vi "DG Do Single Measurement.vi"(6 "Iteration index":i32, 7 "TWM handle in":i32, 8 "error in (no error)":errorcluster, 9 "DG measurement":T1={"Signal frequencies (Hz)"=[1000.0], "Signal amplitudes (V)"=[0.707], "Sampling frequencies (Hz)"=[10000000.0], "Record lengths (multiples of periods)"=[10000.0], "Calculate results"=FALSE, "Algorithm"="TWM-PJVSSubS", "TWM data directories"=[], "TWM data directories relative"=[], "PJVS frequencies (Hz)"=[1000.0], "PJVS reference voltages array of vector cluster"=[], "Requested PJVS steps"=[20], "Data folder"=path "", "Rs"=0, "Re"=0, "Settle down after PJVS change (s)"=1.0, "Switch position"=0.0, "PJVS amplitudes (Hz)"=[1000.0], "DG measurement info files"=[]} {"PJVS amplitudes (Hz)" format="%#_3p"; "PJVS reference voltages array of vector cluster"."PJVS reference voltages vector" format="%#_3p"; "PJVS frequencies (Hz)" format="%#_3p"; "Record lengths (multiples of periods)" format="%#_3p"; "Sampling frequencies (Hz)" format="%#_3p"; "Signal amplitudes (V)" format="%#_3p"; "Signal frequencies (Hz)" format="%#_3p"}, 10 "Common properties":T2={"Measurement status ref"=refnum, "TWM Status ref"=refnum, "Abort ref"=refnum, "Skip waiting ref"=refnum, "GNU Octave path"=path "C:/Program Files/GNU Octave/Octave-6.2.0/mingw64/bin", "TWM+QWTB path"=path "C:/Users/labina/Desktop/TWM-1.8.7.0-full/octprog", "lvlib path"=path "D:/martin/WAC/WACsw - github/control_software/Filter function meter/external libraries/GOLPI 0.7.3.1 source distribution LV 20.0 32 bit/lv_proc.dll", "TWM pipe"="\\\\.\\pipe\\TWM:server", "PJVS status ref"=refnum, "WAC path"=path ""}) -> (0 "error out":errorcluster, 2 "TWM result as number":dbl[][](array[numeric]), 5 "TWM handle out":i32)   [LabVIEW 2020]
doc: "Setup TWM for single CE measurement, start TWM and read output."
uses:
  Utilities/Type definitions/Sampling properties.ctl
  Utilities/Type definitions/Common properties.ctl
  DG measurement.ctl
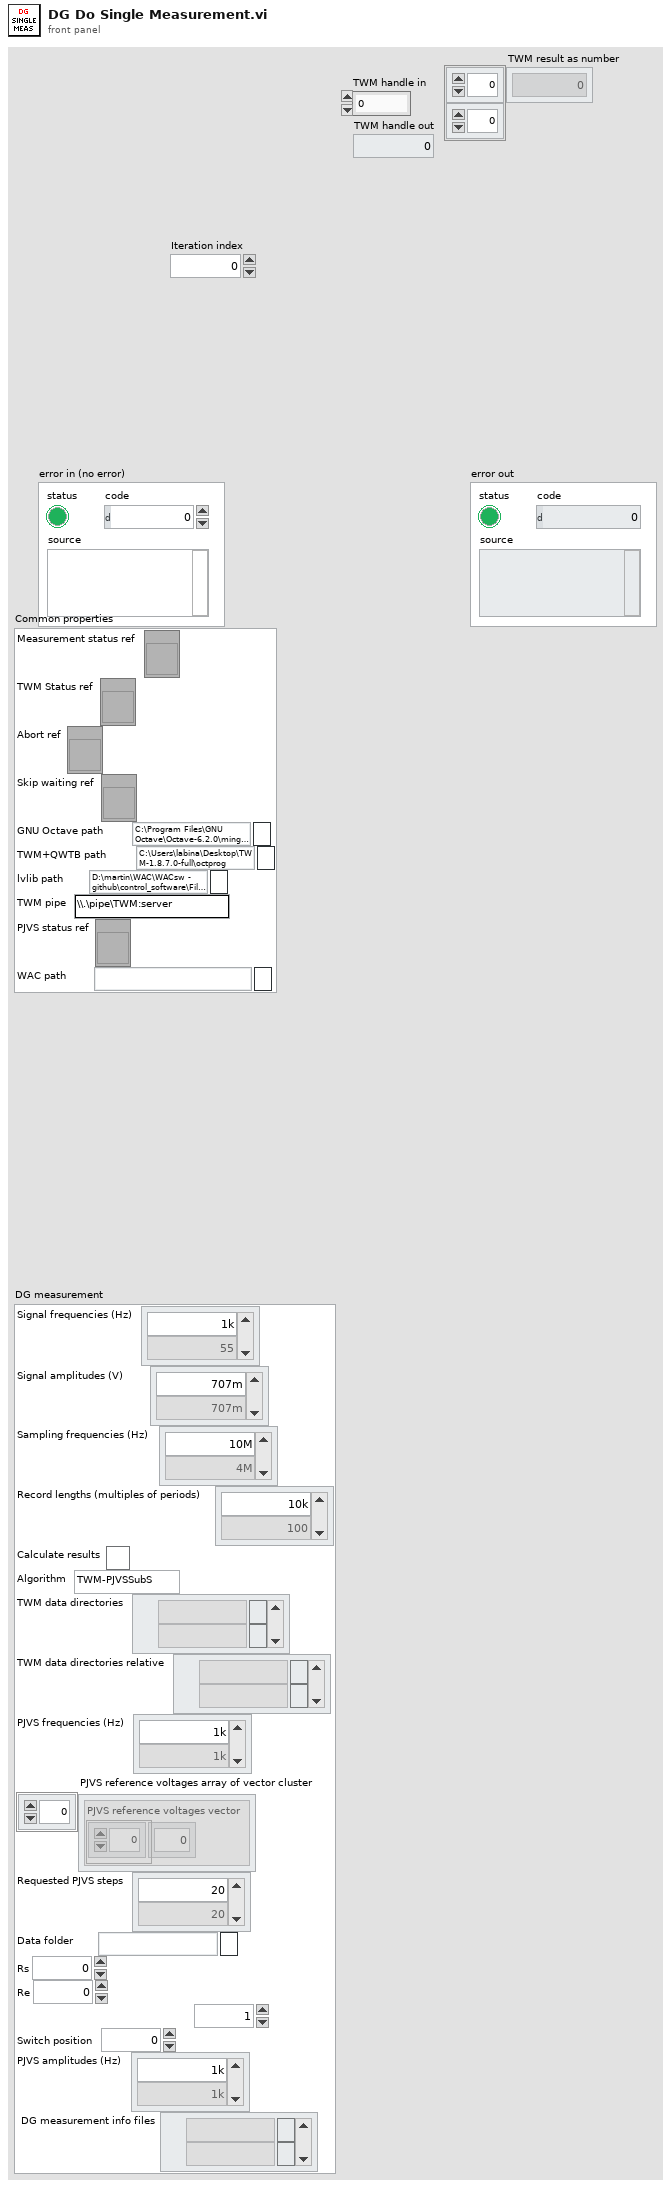
[diagram p1: front panel]
types:
  T1 = typedef "DG measurement.ctl" = cluster{"Signal frequencies (Hz)":dbl[], "Signal amplitudes (V)":dbl[], "Sampling frequencies (Hz)":dbl[], "Record lengths (multiples of periods)":dbl[], "Calculate results":bool, "Algorithm":string, "TWM data directories":path[], "TWM data directories relative":path[], "PJVS frequencies (Hz)":dbl[], "PJVS reference voltages array of vector cluster":cluster{"PJVS reference voltages vector":dbl[]}[], "Requested PJVS steps":u32[], "Data folder":path, "Rs":i32, "Re":i32, "Settle down after PJVS change (s)":dbl, "Switch position":dbl, "PJVS amplitudes (Hz)":dbl[], "DG measurement info files":path[]}
  T2 = typedef "Common properties.ctl" = cluster{"Measurement status ref":refnum<vi>, "TWM Status ref":refnum<vi>, "Abort ref":refnum<vi>, "Skip waiting ref":refnum<vi>, "GNU Octave path":path, "TWM+QWTB path":path, "lvlib path":path, "TWM pipe":string, "PJVS status ref":refnum<vi>, "WAC path":path}
  T3 = typedef "Sampling properties.ctl" = cluster{"Sampling frequency (Hz)":dbl, "Record length (multiples of period)":dbl, "Signal amplitude (V)":dbl, "Measurement frequency (Hz)":dbl, "Calculate RMS from samples":bool, "Algorithm":string, "Measurement path":string}
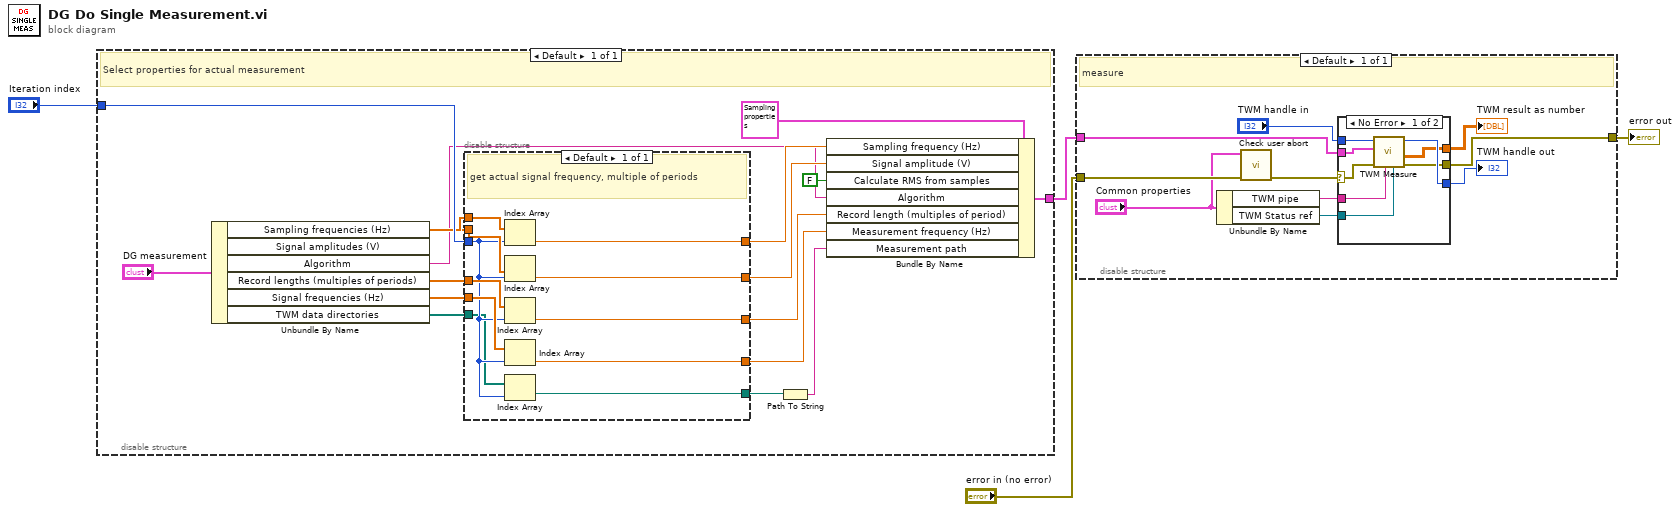
[diagram p0: block diagram]
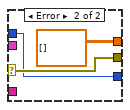
[diagram p2: hidden frame]
diagram:
  n1 = disable-structure shown="Default" {
    disable-tunnel: "Iteration index" -> [w18]
    disable-tunnel: [w19] -> w4
    frame Enabled {
      # "Select properties for actual measurement"
      n2 = Unbundle By Name("DG measurement") -> ("Sampling frequencies (Hz)"=w14:dbl[], "Signal amplitudes (V)"=w13:dbl[], "Algorithm"=w12:string, "Record lengths (multiples of periods)"=w11:dbl[], "Signal frequencies (Hz)"=w10:dbl[], "TWM data directories"=w9:path[])
      n3 = disable-structure shown="Default" {
        disable-tunnel: w10 -> [w32]
        disable-tunnel: w11 -> [w31]
        disable-tunnel: w18 -> [w24]
        disable-tunnel: [w30] -> w17
        disable-tunnel: [w29] -> w21
        disable-tunnel: w13 -> [w28]
        disable-tunnel: [w27] -> w16
        disable-tunnel: w14 -> [w26]
        disable-tunnel: [w25] -> w15
        disable-tunnel: [w22] -> w6
        disable-tunnel: w9 -> [w23]
        frame Enabled {
          # "get actual signal frequency, multiple of periods"
          n4 = Index Array(array=w26, index=w24) -> (element=w25:dbl)
          n5 = Index Array(array=w28, index=w24) -> (element=w27:dbl)
          n6 = Index Array(array=w31, index=w24) -> (element=w29:dbl)
          n7 = Index Array(array=w32, index=w24) -> (element=w30:dbl)
          n8 = Index Array(array=w23, index=w24) -> (element=w22:path)
        }
      }
      n9 = Path To String(path=w6) -> (string=w5:string)
      n10 = Bundle By Name(cluster=T3 {"Sampling frequency (Hz)"=500000.0, "Record length (multiples of period)"=1000.0, "Signal amplitude (V)"=4.5, "Measurement frequency (Hz)"=1000.0, "Calculate RMS from samples"=FALSE, "Algorithm"="TWM-WFFT", "Measurement path"=""} ("TWM Measurement properties"), "Sampling frequency (Hz)"=w15, "Signal amplitude (V)"=w16, "Calculate RMS from samples"=FALSE, "Algorithm"=w12, "Record length (multiples of period)"=w21, "Measurement frequency (Hz)"=w17, "Measurement path"=w5) -> (w19:T3)
    }
  }
  n11 = disable-structure shown="Default" {
    disable-tunnel: "error in (no error)" -> [w42]
    disable-tunnel: [w35] -> w3
    disable-tunnel: w4 -> [w41]
    frame Enabled {
      # "measure"
      n12 = Unbundle By Name("Common properties") -> ("TWM pipe"=w39:string, "TWM Status ref"=w38:refnum<vi>)
      n13 = call "Check user abort.vi"("error in (no error)"=w42, "Common properties"="Common properties") -> ("error out"=w33:errorcluster)  [unwired: 9 in]
      n14 = case shown="No Error" w33 {
        selector: w33 -> [w43 w53]
        tunnel: w41 -> [w50 _]
        tunnel: w39 -> [w49 _]
        tunnel: w38 -> [w48 _]
        tunnel: "TWM handle in" -> [w47 w52]
        tunnel: [w46 w52] -> w36
        tunnel: [w45 w53] -> w35
        tunnel: [w44 dbl[][] [] ("TWM result as number")] -> w34
        frame No Error {
          n15 = call "TWM Measure.vi"("TWM Status ref"=w48, "TWM pipe"=w49, "error in (no error)"=w43, "TWM Measurement properties"=w50, "TWM handle"=w47) -> ("error out"=w45:errorcluster, "TWM result as number"=w44:dbl[][], "TWM handle out"=w46:i32)  [unwired: 3 in, 1 out]
        }
        frame Error {
        }
      }
      "TWM handle out" <- w36
      "TWM result as number" <- w34
    }
  }
  "error out" <- w3
